vi "[Global] Template.vi"() -> ()   [LabVIEW 2019]
uses:
  <vilib>/vision/Image Controls.llb/IMAQ Image.ctl
panel:
  in  "TemplateArray":T2(array[cluster])
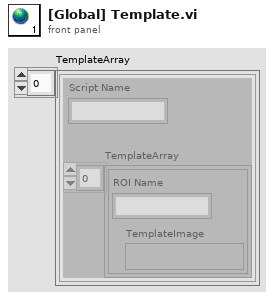
[diagram p1: front panel]
types:
  T1 = typedef "IMAQ Image.ctl" = refnum<image>
  T2 = cluster{"Script Name":string, "TemplateArray":cluster{"ROI Name":string, "TemplateImage":T1}[]}[]
diagram:
